vi "GuiPanelClose.vi"(8 "error in (no error)":errorcluster, 11 "GuiInterface in":refnum<class "GuiInterface.lvclass">) -> (0 "error out":errorcluster, 3 "GuiInterface out":refnum<class "GuiInterface.lvclass">)   [LabVIEW 2022 SP3, in "Test.lvlib" / "Gui.lvlib" / "GuiInterface.lvclass"]
uses:
  GuiInterface.lvclass
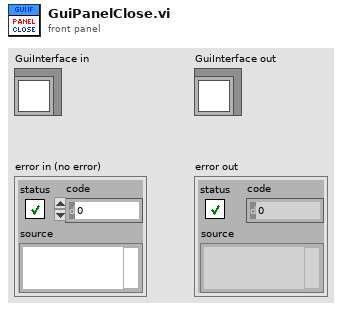
[diagram p1: front panel]
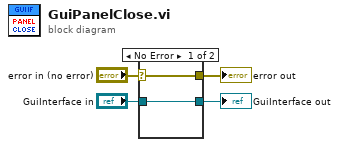
[diagram p0: block diagram]
diagram:
  n1 = case shown="No Error" "error in (no error)" {
    selector: "error in (no error)" -> [w5 w8]
    tunnel: [w5 w8] -> w3
    tunnel: [w6 w7] -> w1
    tunnel: "GuiInterface in" -> [w6 w7]
    frame No Error {
    }
    frame Error {
    }
  }
  "error out" <- w3
  "GuiInterface out" <- w1
